vi "Filter Targets.vi"(9 "Bank":u32[](array[numeric]), 11 "Names":string[](array[string])) -> (1 "Bank 2":string[](array[string]), 3 "Bank 1":string[](array[string]))   [LabVIEW 2019, in "MLTFNC.lvlib" / "MLTFNC.lvclass"]
uses:
  Library/MLTFNC.lvclass
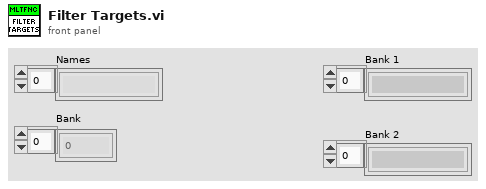
[diagram p1: front panel]
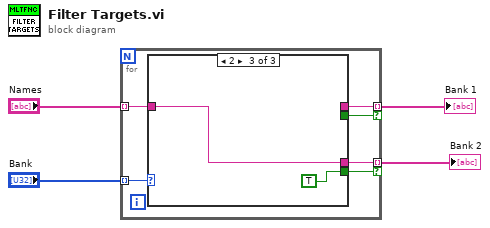
[diagram p0: block diagram]
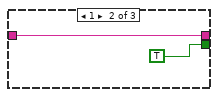
[diagram p3: hidden frame]
diagram:
  n1 = for {
    tunnel: "Names" -> [w9] mode=indexing
    tunnel: "Bank" -> [w10] mode=indexing
    tunnel: [w8] -> w1 mode=indexing if=w7
    tunnel: [w6] -> w2 mode=indexing if=w5
    n2 = case shown="2" w10 {
      tunnel: w9 -> [_ w12 w14]
      tunnel: [_ w12 _] -> w8
      tunnel: [_ TRUE _] -> w7
      tunnel: [_ _ w14] -> w6
      tunnel: [_ _ TRUE] -> w5
      frame Default {
      }
      frame 1 {
      }
      frame 2 {
      }
    }
  }
  "Bank 1" <- w1
  "Bank 2" <- w2
